vi "Close.vi"(8 "error in (no error)":errorcluster caption="错误输入（无错误）", 11 "VISA资源名称":refnum<visa-resource-name>) -> (0 "错误输出":errorcluster)   [LabVIEW 2018]
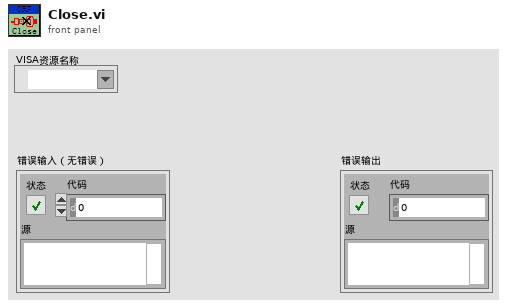
[diagram p1: front panel]
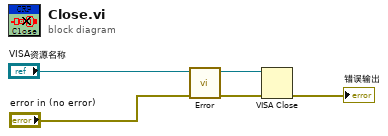
[diagram p0: block diagram]
diagram:
  n1 = call "Error.vi"("error in (no error)"="error in (no error)", "VISA资源名称"="VISA资源名称") -> ("错误输出"=w2:errorcluster, "VISA引用句柄输出"=w3:refnum<visa-resource-name>)  [unwired: 6 in, 2 out]
  n2 = VISA Close(VISA resource name=w3, error in (no error)=w2) -> (error out=→"错误输出":errorcluster)
